vi "MM6.PG_ShiftChannels_HyperKnorz.vi"(9 "patternNumber":i32, 10 "PatternTable":string[](array[string])) -> (2 "PatternTableShifted":string[](array[string]))   [LabVIEW 2014, in "MM6.lvlib"]
doc: "Shifts the channels for each patternTable by 16 channels times the number of the pattern. This is a hyper-knorz solution, to achieve that all 48 channels of the PPG card can be used, although the GUI supports only 16 channels."
uses:
  MM6.lvlib
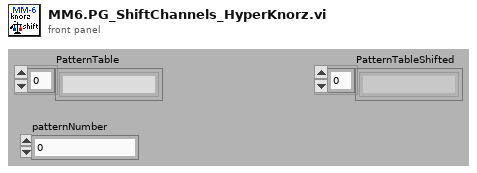
[diagram p1: front panel]
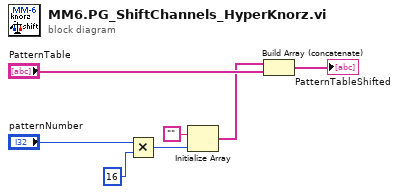
[diagram p0: block diagram]
diagram:
  n1 = Multiply(x="patternNumber", y=16 ("dimension size")) -> (x*y=w5:i32)
  n2 = Initialize Array("", w5) -> (w2:string[])
  n3 = Build Array (concatenate)(w2, "PatternTable") -> (→"PatternTableShifted":string[])
